vi "TestSpeedProfileCreation.vi"() -> ()   [LabVIEW 2017]
uses:
  <vilib>/addons/InsightCM/Devices/Shared/VibrationVirtualChannel/controls/FixedSpeed.ctl
  <vilib>/addons/InsightCM/Utilities/Analysis/Shared/AnalysisHelper.lvlib
  <vilib>/addons/InsightCM/Devices/Shared/AcquireBaseLoop/controls/PulsePositions.ctl
panel:
  in  "Blocks to Process":i32=5
  out "Total Pulses":i32
  out "Pulses Per Block":dbl
  in  "Speed Ratio":dbl=1.0
  in  "Nominal Speed":dbl=3600.0
  out "Pulse Spacing Identical":bool
  out "Speeds Match":bool
  out "Pulse Positions":T1[](array[typedef])
  out "speed (calculated)":dbl
  out "Waveform Graph":dbl[](graph)
  out "Array 3":dbl[](array[numeric])
  out "min pulse spacing":dbl
  out "max pulse spacing":dbl
  out "Fixed Speed Configs":T2[](array[typedef])
  # "These max and min values should be equal"
  # "This graph should be a straight line"
  # "This speed should equal the\nNominal Speed control above"
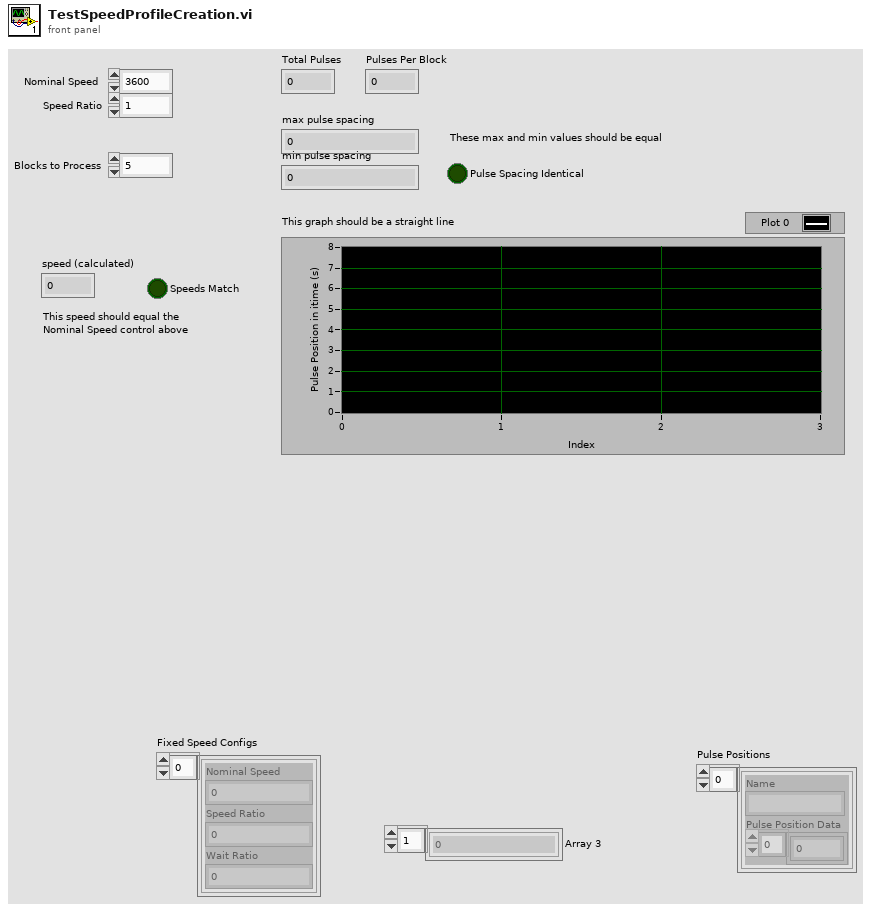
[diagram p1: front panel]
types:
  T1 = typedef "PulsePositions.ctl" = cluster{"Name":string, "Pulse Position Data":dbl[]}
  T2 = typedef "VibrationVirtualChannel.lvlib/FixedSpeed.ctl" = cluster{"Nominal Speed":dbl, "Speed Ratio":dbl, "Wait Ratio":dbl}
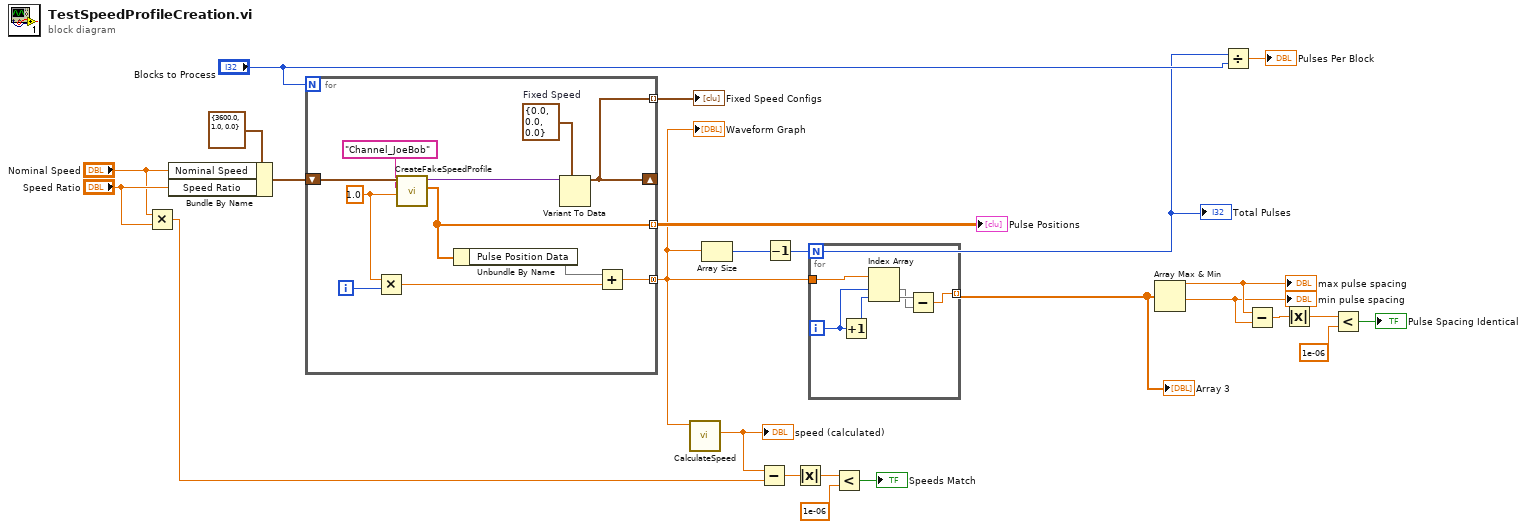
[diagram p0: block diagram]
diagram:
  n1 = Multiply(x="Nominal Speed", y="Speed Ratio") -> (x*y=w3:dbl)
  n2 = Bundle By Name(cluster=T2 {"Nominal Speed"=3600.0, "Speed Ratio"=1.0, "Wait Ratio"=0.0} ("Fixed Speed"), "Nominal Speed"="Nominal Speed", "Speed Ratio"="Speed Ratio") -> (w10:T2)
  n3 = for {
    N: "Blocks to Process" -> [_]
    tunnel: [w30] -> w22 mode=indexing
    shift-right: [w31] -> _
    shift-left: w10 -> [w35]
    tunnel: [w31] -> w24 mode=indexing
    tunnel: [w25] -> w7 mode=concatenating
    i -> [w28]
    w33 = T2 {"Nominal Speed"=0.0, "Speed Ratio"=0.0, "Wait Ratio"=0.0}  # Fixed Speed
    w27 = 1.0 ("Block Size (s)")
    n4 = Multiply(x=w27, y=w28) -> (x*y=w26:dbl)
    n5 = call <vilib>:"CreateFakeSpeedProfile.vi"("block size (s)"=w27, 10:"Channel_JoeBob" ("Channel Name"), "fixed speed config in"=w35) -> ("pulse positions"=w30:dbl[], "fixed speed config out"=w32:variant)  [unwired: 5 in, 2 out]
    n6 = Unbundle By Name(w30) -> ("Pulse Position Data"=w29)
    n7 = Variant To Data(type=w33, Variant=w32) -> (data=w31:T2)  [unwired: 1 in, 1 out]
    n8 = Add(x=w29, y=w26) -> (x+y=w25:dbl)
  }
  "Fixed Speed Configs" <- w24
  "Waveform Graph" <- w7
  "Pulse Positions" <- w22
  n9 = call <vilib>:"CalculateSpeed.vi"("Pulse Positions"=w7) -> ("Speed (RPM)"=w6:dbl)  [unwired: 9 in, 1 out]
  "speed (calculated)" <- w6
  n10 = Array Size(array=w7) -> (size(s)=w2:i32)
  "Total Pulses" <- w2
  n11 = Subtract(x=w6, y=w3) -> (x-y=w15:dbl)
  n12 = Decrement(x=w2) -> (x-1=w1:i32)
  n13 = Absolute Value(x=w15) -> (abs(x)=w14:dbl)
  n14 = for {
    N: w1 -> [_]
    tunnel: w7 -> [w41]
    tunnel: [w38] -> w23 mode=indexing
    i -> [w39]
    n15 = Increment(x=w39) -> (x+1=w40:i32)
    n16 = Index Array(array=w41, index #1=w39, index #2=w40) -> (element #1=w36, element #2=w37)
    n17 = Subtract(x=w37, y=w36) -> (x-y=w38:dbl)
  }
  "Array 3" <- w23
  n18 = Less?(x=w14, y=1e-06) -> (x < y?=→"Speeds Match":bool)
  n19 = Array Max & Min(array=w23) -> (max value=w17:dbl, min value=w16:dbl)  [unwired: 2 out]
  "max pulse spacing" <- w17
  "min pulse spacing" <- w16
  n20 = Divide(x=w2, y="Blocks to Process") -> (x/y=→"Pulses Per Block":dbl)
  n21 = Subtract(x=w17, y=w16) -> (x-y=w13:dbl)
  n22 = Absolute Value(x=w13) -> (abs(x)=w12:dbl)
  n23 = Less?(x=w12, y=1e-06) -> (x < y?=→"Pulse Spacing Identical":bool)
